vi "Generate System Integrity File.vi"(0 "System Integrity File Path":path, 1 "File Paths":path[](array[path]), 2 "System Key":string, 3 "USER_NAME":string, 5 "Error In":errorcluster) -> (19 "Error Out":errorcluster)   [LabVIEW 2010]
doc: "This VI writes a System Integrity File. The Array input lists the Package Integrity Files to include in this file. The System Key is used to encrypt the internal integrity string.\n\nCurrent Revision: 17\nVSS Version: 7\nCopyright 2002 VI Engineering, Inc."
uses:
  <vilib>/Utility/config.llb/NI_LVConfig.lvlib
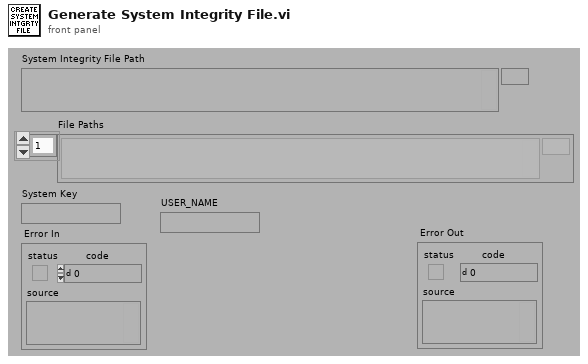
[diagram p1: front panel]
types:
  T1 = typedef "NI_LVConfig.lvlib/Config Data RefNum.ctl" = refnum<k1>
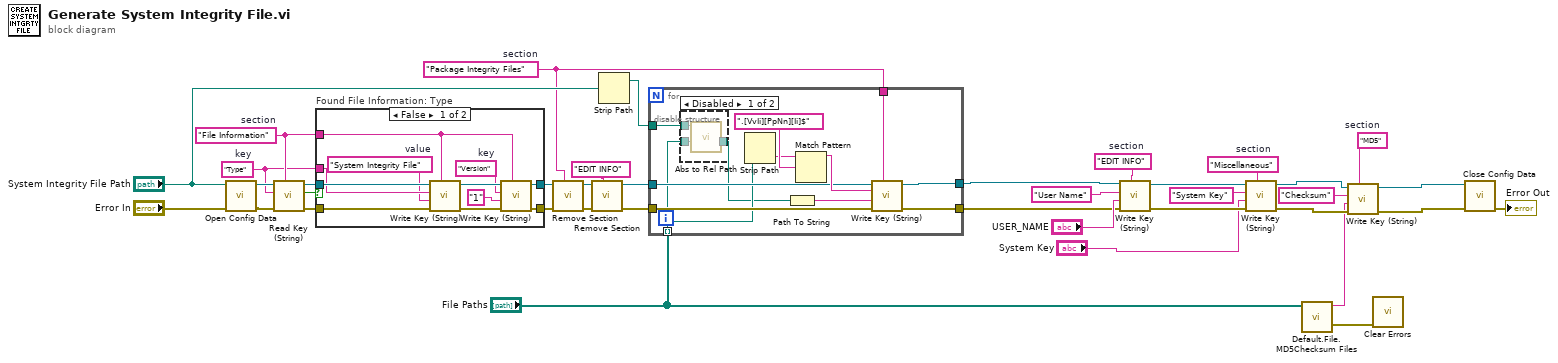
[diagram p0: block diagram]
diagram:
  w8 = "MD5"  # section
  w18 = "Miscellaneous"  # section
  w19 = "EDIT INFO"  # section
  w26 = "Package Integrity Files"  # section
  w31 = "Type"  # key
  w32 = "File Information"  # section
  n1 = call <vilib>:"Open Config Data.vi"("error in (no error)"="Error In", "configuration file path"="System Integrity File Path") -> ("error out"=w36:errorcluster, "refnum"=w37:T1)  [unwired: 7 in, 1 out]
  n2 = call <vilib>:"Read Key (String).vi"("section"=w32, "error in (no error)"=w36, "key"=w31, "refnum"=w37) -> ("error out"=w33:errorcluster, "found?"=w35:bool, "refnum out"=w34:T1)  [unwired: 4 in, 1 out]
  n3 = case "Found File Information: Type" shown="False" w35 {
    tunnel: w34 -> [w49 w51]
    tunnel: w33 -> [w48 w50]
    tunnel: w32 -> [w41 _]
    tunnel: w31 -> [w47 _]
    tunnel: [w44 w51] -> w28
    tunnel: [w43 w50] -> w27
    frame False {
      w40 = "Version"  # key
      w46 = "System Integrity File"  # value
      n4 = call <vilib>:"Write Key (String).vi"("section"=w41, "error in (no error)"=w48, "value"=w46, "key"=w47, "refnum"=w49) -> ("error out"=w42:errorcluster, "refnum out"=w45:T1)  [unwired: 4 in, 1 out]
      n5 = call <vilib>:"Write Key (String).vi"("section"=w41, "error in (no error)"=w42, "value"="1", "key"=w40, "refnum"=w45) -> ("error out"=w43:errorcluster, "refnum out"=w44:T1)  [unwired: 4 in, 1 out]
    }
    frame True {
      # "The section exists. No need to write to this section."
    }
  }
  n6 = call <vilib>:"Remove Section.vi"("section"=w26, "error in (no error)"=w27, "refnum"=w28) -> ("error out"=w23:errorcluster, "refnum out"=w25:T1)  [unwired: 6 in, 1 out]
  n7 = call <vilib>:"Remove Section.vi"("section"="EDIT INFO", "error in (no error)"=w23, "refnum"=w25) -> ("error out"=w22:errorcluster, "refnum out"=w24:T1)  [unwired: 6 in, 1 out]
  n8 = Strip Path(path="System Integrity File Path") -> (stripped path=w29:path)  [unwired: 1 out]
  n9 = for {
    tunnel: [w61] -> w12
    tunnel: [w60] -> w11
    tunnel: w24 -> [w59]
    tunnel: w22 -> [w58]
    tunnel: "File Paths" -> [w55] mode=indexing
    tunnel: w29 -> [w57]
    tunnel: w26 -> [w54]
    n10 = disable-structure shown="Disabled" {
      disable-tunnel: w57 -> [w66 _]
      disable-tunnel: w55 -> [w65 w67]
      disable-tunnel: [w64 w67] -> w53
      frame Disabled {
        n11 = call "Abs to Rel Path.vi"("File Path"=w65, "Base Path"=w66) -> ("Path Out"=w64:path)  [unwired: 8 in, 1 out]
      }
      frame Enabled {
      }
    }
    n12 = Strip Path(path=w55) -> (name=w56:string)  [unwired: 1 out]
    n13 = Path To String(path=w53) -> (string=w52:string)
    n14 = Match Pattern(string=w56, regular expression=".[VvIi][PpNn][Ii]$") -> (before substring=w63:string)  [unwired: 1 in, 3 out]
    n15 = call <vilib>:"Write Key (String).vi"("section"=w54, "error in (no error)"=w58, "value"=w52, "key"=w63, "refnum"=w59) -> ("error out"=w60:errorcluster, "refnum out"=w61:T1)  [unwired: 4 in, 1 out]
  }
  n16 = call <vilib>:"Write Key (String).vi"("section"=w19, "error in (no error)"=w11, "value"="USER_NAME", "key"="User Name", "refnum"=w12) -> ("error out"=w15:errorcluster, "refnum out"=w16:T1)  [unwired: 4 in, 1 out]
  n17 = call <vilib>:"Write Key (String).vi"("section"=w18, "error in (no error)"=w15, "value"="System Key", "key"="System Key", "refnum"=w16) -> ("error out"=w5:errorcluster, "refnum out"=w7:T1)  [unwired: 4 in, 1 out]
  n18 = call "Default.File.MD5Checksum Files.vi"("FilePaths"="File Paths") -> ("error out"=w3:errorcluster, "MD5 message-digest"=w2:string)  [unwired: 8 in, 1 out]
  n19 = call <vilib>:"Write Key (String).vi"("section"=w8, "error in (no error)"=w5, "value"=w2, "key"="Checksum", "refnum"=w7) -> ("error out"=w4:errorcluster, "refnum out"=w6:T1)  [unwired: 4 in, 1 out]
  n20 = call <vilib>:"Clear Errors.vi"("error in (no error)"=w3) -> ()  [unwired: 6 in, 1 out]
  n21 = call <vilib>:"Close Config Data.vi"("error in (no error)"=w4, "refnum"=w6) -> ("error out"=→"Error Out":errorcluster)  [unwired: 8 in, 1 out]
